vi "Main.vi"() -> ()   [LabVIEW 2018]
uses:
  ScintillaNET.dll
panel:
  in  "Scintilla":refnum<k24>(container)
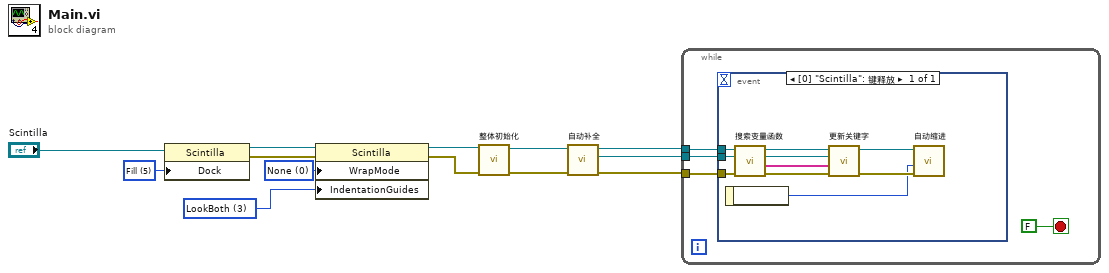
[diagram p0: block diagram]
diagram:
  w10 = 3 items=["None", "Real", "LookForward", "LookBoth"] ("IndentationGuides")
  w11 = 0 items=["None", "Word", "Char", "Whitespace"] ("WrapMode")
  w12 = 5 items=["None", "Top", "Bottom", "Left", "Right", "Fill"] ("Dock")
  n1 = property class="Scintilla"(reference="Scintilla", "Dock"=w12) -> (reference out=w9:refnum<k24>, error out=w8:errorcluster)  [unwired: 1 in]
  n2 = property class="Scintilla"(reference=w9, error in=w8, "WrapMode"=w11, "IndentationGuides"=w10) -> (reference out=w1:refnum<k24>, error out=w13:errorcluster)
  n3 = call "整体初始化.vi"("错误输入（无错误）"=w13, "Scintilla"=w1) -> ("错误输出"=w7:errorcluster, "引用输出"=w4:refnum<k24>)  [unwired: 8 in]
  n4 = call "自动补全.vi"("错误输入"=w7, "引用"=w4) -> ("错误输出"=w6:errorcluster, "引用输出 2"=w5:refnum<k24>, "引用输出"=w3:refnum<k24>)  [unwired: 7 in]
  n5 = while {
    tunnel: w3 -> [w14]
    tunnel: w6 -> [w15]
    tunnel: w5 -> [w16]
    stop <- FALSE stop-if-true
    n6 = event shown="[0] \"Scintilla\": 键释放" {
      selector: _ -> [_]
      dyn-events: _ -> [_]
      timeout: _ -> [_]
      tunnel: w16 -> [w26]
      tunnel: w15 -> [w25]
      tunnel: w14 -> [w24]
      event "Scintilla": Key Up {
        n7 = event-data() -> ("ScanCode"=w18:i16)  [unwired: 1 in]
        n8 = call "搜索变量函数.vi"("错误输入"=w25, "引用"=w24) -> ("错误输出"=w21:errorcluster, "输出数组"=w23:string[], "引用输出"=w22:refnum<k24>)  [unwired: 7 in]
        n9 = call "更新关键字.vi"("错误输入"=w21, "变量函数"=w23, "引用 2"=w26, "引用"=w22) -> ("错误输出"=w19:errorcluster, "引用输出"=w20:refnum<k24>)  [unwired: 5 in, 1 out]
        n10 = call "自动缩进.vi"("错误输入"=w19, "扫描代码"=w18, "引用"=w20) -> ()  [unwired: 7 in, 2 out]
      }
    }
  }
